vi "ArrayAnalysis.vi"(10 "Numeric":i32, 11 "Array in":dbl[](array[numeric])) -> (3 "Array out":dbl[](array[numeric]))   [LabVIEW 2011]
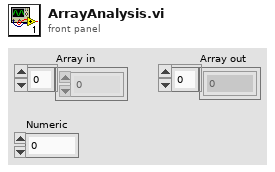
[diagram p1: front panel]
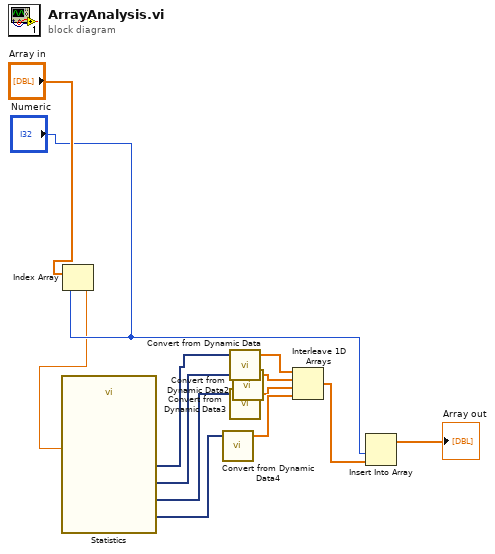
[diagram p0: block diagram]
diagram:
  n1 = Index Array(array="Array in", index="Numeric") -> (element=w1:dbl)
  n2 = call "Statistics"("Signals"=w1) -> ("Median"=w4:dynamicdata, "Variance"=w5:dynamicdata, "Minimum"=w2:dynamicdata, "Maximum"=w3:dynamicdata)  [unwired: 22 in, 1 out]
  n3 = call "Convert from Dynamic Data4"("Dynamic Data Type"=w2) -> ("Array"=w9:dbl[])  [unwired: 3 in]
  n4 = call "Convert from Dynamic Data"("Dynamic Data Type"=w5) -> ("Array"=w6:dbl[])  [unwired: 3 in]
  n5 = call "Convert from Dynamic Data3"("Dynamic Data Type"=w3) -> ("Array"=w8:dbl[])  [unwired: 3 in]
  n6 = call "Convert from Dynamic Data2"("Dynamic Data Type"=w4) -> ("Array"=w7:dbl[])  [unwired: 3 in]
  n7 = Interleave 1D Arrays(w6, w7, w8, w9) -> (w10:dbl[])
  n8 = Insert Into Array(index="Numeric", new element=w10) -> (→"Array out":dbl[])  [unwired: 1 in]
